vi "Init Events.vi"(8 "error in (no error)":errorcluster, 11 "CoolApp in":refnum<class "CoolApp.lvclass">) -> (0 "error out":errorcluster, 3 "CoolApp out":refnum<class "CoolApp.lvclass">)   [LabVIEW 2020, in "LAF2024Q2.lvlib" / "CoolApp.lvclass"]
uses:
  CoolApp.lvclass
  State Update.ctl
  Nested.ctl
  Process State.ctl
  CoolApp.lvclass/CoolApp.ctl
  LAF2024Q2.lvlib
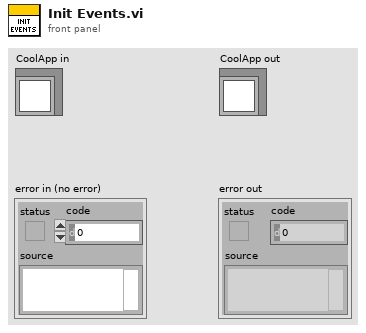
[diagram p1: front panel]
types:
  T1 = typedef "LAF2024Q2.lvlib/CoolApp.lvclass/State Update.ctl" = cluster{"Nested":T2, "Process State":T3}
  T2 = typedef "LAF2024Q2.lvlib/CoolApp.lvclass/Nested.ctl" = enum16{"DAQ", "Chart"}
  T3 = typedef "LAF2024Q2.lvlib/Process State.ctl" = enum16{"Idle", "Initializing", "Starting", "Running", "Stopping", "Stopped"}
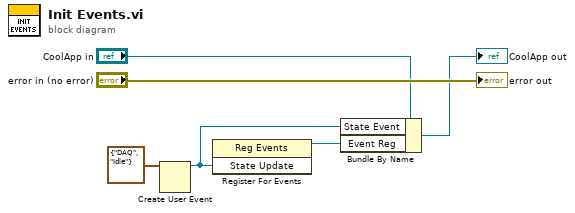
[diagram p0: block diagram]
diagram:
  n1 = Create User Event(user event datatype=T1 {"Nested"=enum."DAQ", "Process State"=enum."Idle"} ("State Update")) -> (user event=w3:refnum<user-event>)  [unwired: 1 in, 1 out]
  n2 = register-events(w3) -> (reference out=w4:refnum<event-registration>)  [unwired: 2 in, 1 out]
  n3 = Bundle By Name(cluster="CoolApp in", "State Event"=w3, "Event Reg"=w4) -> (→"CoolApp out":refnum<class "CoolApp.lvclass">)
  "error out" <- "error in (no error)"
